vi "Radio Frequency Identification.vi"(0 "LINX Resource":T1, 5 "RFID Value":u8[](array[numeric]), 11 "Error In":errorcluster) -> (4 "LINX Resource Out":T1, 6 "Response":u8[](array[numeric]), 8 "Wrong ID":bool, 10 "Correct ID":bool, 15 "Error Out":errorcluster)   [LabVIEW 2020]
doc: "Determines whether \"RFID Value\" is found. If found then \"Correc ID\" is true and \"Wrong ID\" is false. If another RFID value comes in contacted that was not specified by \"RFID Value\" then \"Wrong ID\" is true and \"Correct ID\" is false. If no RFID comes in contact then both \"Wrong ID\" and \"Correct ID\" are false."
uses:
  <vilib>/MakerHub/LINX/Private/Type Defs/LINX Ref.ctl
  <vilib>/MakerHub/LINX/Private/Type Defs/Platform.ctl
  <vilib>/MakerHub/LINX/Private/Type Defs/Interface.ctl
  <vilib>/MakerHub/LINX/Private/Device/Type Defs/LINX Device Config.ctl
  <vilib>/MakerHub/LINX/Private/Device/Type Defs/TCP Config.ctl
  <vilib>/MakerHub/LINX/Private/Device/Type Defs/Channels.ctl
  <vilib>/MakerHub/LINX/LMH-LINX.lvlib
  <vilib>/MakerHub/LINX/Private/Device/Device.lvlib
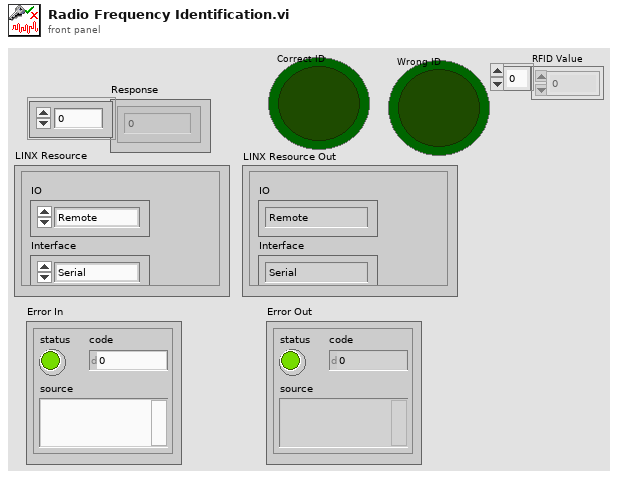
[diagram p1: front panel]
types:
  T1 = typedef "LMH-LINX.lvlib/LINX Ref.ctl" = cluster{"IO":T2, "Interface":T3, "LINX Device Config":T4}
  T2 = typedef "LMH-LINX.lvlib/Platform.ctl" = enum16{"Remote", "Local"}
  T3 = typedef "LMH-LINX.lvlib/Interface.ctl" = enum16{"Serial", "TCP"}
  T4 = typedef "LMH-LINX.lvlib/Device.lvlib/LINX Device Config.ctl" = cluster{"Interface":T3, "COM Port":refnum<visa-resource-name>, "TCP Configuration":T5, "Device Family":u8, "Device ID":u8, "Device Name":string, "TCP Ref":refnum<k5>, "Channels":T6}
  T5 = typedef "LMH-LINX.lvlib/Device.lvlib/TCP Config.ctl" = cluster{"IP Address":string, "Port":u16}
  T6 = typedef "LMH-LINX.lvlib/Channels.ctl" = cluster{"DI":u8[], "DO":u8[], "AI":u8[], "AO":u8[], "PWM":u8[], "QE":u8[], "UART":u8[], "I2C 2":u8[], "SPI":u8[], "CAN":u8[], "Servo":u8[], "AI Ref (V)":dbl, "AI Resolution (Bits)":u8, "AO Ref (V)":dbl, "AO Resolution (Bits)":u8}
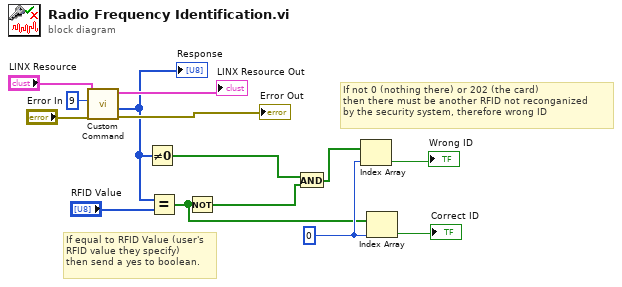
[diagram p0: block diagram]
diagram:
  w6 = 0 ("index")
  # "If not 0 (nothing there) or 202 (the card)\nthen there must be another RFID not reconganized \nby the security system, therefore wrong ID"
  # "If equal to RFID Value (user's\nRFID value they specify)\nthen send a yes to boolean."
  n1 = call <vilib>:"Custom Command.vi"("Error In"="Error In", "Custom Command Number"=u16 9, "LINX Resource"="LINX Resource") -> ("Error Out"=→"Error Out":errorcluster, "Response"=w9:u8[], "LINX Resource"=→"LINX Resource Out":T1)  [unwired: 5 in, 1 out]
  "Response" <- w9
  n2 = Not Equal To 0?(x=w9) -> (x != 0?=w8:bool[])
  n3 = Equal?(x=w9, y="RFID Value") -> (x = y?=w3:bool[])
  n4 = Not(x=w3) -> (.not. x?=w4:bool[])
  n5 = And(x=w8, y=w4) -> (x .and. y?=w7:bool[])
  n6 = Index Array(array=w7, index=w6) -> (element=→"Wrong ID":bool)
  n7 = Index Array(array=w3, index=w6) -> (element=→"Correct ID":bool)
